vi "Keithley24XX_SR830_PPMS6000_4Probe_Resistance_Measurement - MasterSlave.vi"() -> ()   [LabVIEW 2019]
uses:
  <instrlib>/Stanford Research 830/Public/Data/Read (All Parameters).vi
  <instrlib>/Keithley 24XX/Public/Data/Read (Single Point).vi
  <instrlib>/Keithley 24XX/Keithley 24XX.lvlib
  <instrlib>/Stanford Research 830/Stanford Research 830.lvlib
panel:
  in  "Temperature Control":enum32{"XY Graph", "Waveform (Time)"}(tab)
  out "Temp vs Time : XYGraph 3":cluster{"Y":dbl[], "Y":dbl[]}[](graph)
  out "Temp vs Time: TimeGraph 3":cluster{dbl, "Theta-Value":dbl}[](graph)
  in  "PPMS Temp GPIB address":string="15"
  in  "Daugher Theta vs Vg":enum32{"XY Graph", "Waveform (Time)"}(tab)
  out "Parent Theta vs Vg : XYGraph 2":cluster{"Y":dbl[], "Y":dbl[]}[](graph)
  out "Parent: Theta vs Vg : TimeGraph 2":cluster{dbl, "Theta-Value":dbl}[](graph)
  in  "Daughter R vs Vg 2":enum32{"XY Graph", "Waveform (Time)"}(tab)
  out "Daughter Resistance vs Vg : XYGraph 2":cluster{"Y":dbl[], "Y":dbl[]}[](graph)
  out "Daughter: R vs Vg : TimeGraph 2":cluster{dbl, dbl}[](graph)
  out "dup path 2":path
  in  "<File Name>.txt (Don't add extension) 2":string
  in  "Data Save Path: Daughter":path=path "C:/Users/labpc/Documents/ProbeStation Users Data"
  in  "Sensitivity (Initial Value) 2":i16(ring)=17 items=["Auto Gain"=-1, "2 nV/fA"=0, "5 nV/fA"=1, "10 nV/fA"=2, "20 nV/fA"=3, "50 nV/fA"=4, "100 nV/fA"=5, "200 nV/fA"=6, "500 nV/fA"=7, "1 uV/pA"=8, "2 uV/pA"=9, "5 uV/pA"=10, "10 uV/pA"=11, "20 uV/pA"=12, "50 uV/pA"=13, "100 uV/pA"=14, "200 uV/pA"=15, "500 uV/pA"=16, "1 mV/nA"=17, "2 mV/nA"=18, "5 mV/nA"=19, "10 mV/nA"=20, "20 mV/nA"=21, "50 mV/nA"=22, "100 mV/nA"=23, "200 mV/nA"=24, "500 mV/mA"=25, "1 V/uA"=26]
  in  "Dynamic Reserve (-1 = Auto) 2":i16(ring)=1 items=["Auto Reserve"=-1, "High Reserve"=0, "Normal"=1, "Low Noise"=2]
  in  "Input Connection (0: Single-Ended Voltage)  2":u16(ring)=1 items=["Single-Ended Voltage", "Differential Voltage", "1 MOhm Current Gain", "100 MOhm Current Gain"]
  out "Input Coupling (0: AC) 2":u16(ring) items=["AC", "DC"]
  in  "Time Constant (8: 100ms) 2":u16(ring)=11 items=["10 us", "30 us", "100 us", "300 us", "1 ms", "3 ms", "10 ms", "30 ms", "100 ms", "300 ms", "1 s", "3 s", "10 s", "30 s", "100 s", "300 s", "1 ks", "3 ks", "10 ks", "30 ks"]
  in  "SR830 VISA resource name 2":refnum<visa-resource-name>="GPIB0::8::INSTR"
  in  "Trigger Source (0: Start Feature Off, 1: On)  - Data":u16(ring)=1 items=["Internal", "External"]
  out "Manual Phase (0 Degree) 2":dbl
  out "Detection Harmonic Number 2":dbl=1.0
  out "External Reference Trigger (0: Sine Zero Crossing)  2":u16(ring) items=["Sine Zero Crossing", "TTL Rising Edge", "TTL Falling Edge"]
  in  "Internal Reference Frequency (1000 Hz) 2":dbl=17.0
  in  "Reference Source (1: Internal) 2":u16(ring) items=["External", "Internal"]
  in  "Sine Output Amplitude (V) 2":dbl=1.0
  out "Gate\nVoltage":sgl
  out "Status":sgl
  out "Leakage \nCurrent":sgl
  out "dup path":path
  in  "<File Name>.txt (Don't add extension)":string
  in  "Data Save Path: Source":path=path "C:/Users/labpc/Documents/ProbeStation Users Data"
  in  "I_leak vs Vg":enum32{"XY Graph", "Waveform (Time)"}(tab)
  out "I_leak vs Vg : XYGraph":cluster{"Y":dbl[], "Y":dbl[]}[](graph)
  out "I_leak vs Vg : TimeGraph":cluster{dbl, "Current":sgl}[](graph)
  in  "Gate Voltage\nInitial (V)":dbl
  out "Gate Voltage\nTraversal Direction":enum16{"Upward", "Downward"}(ring)
  in  "Series Resistance \n(Apparatus Constant)":dbl=10000000.0
  in  "stop":bool
  out "Max/Min(-) \nGate Voltage (V)":dbl=80.0
  in  "Gate Voltage \nStep Size (V)":dbl=0.1
  in  "High Gate \nVoltage (V)":dbl
  in  "Low Gate \nVoltage (V)":dbl
  out "Compliance\n Level (A)":dbl=0.1
  in  "Parent Theta vs Vg":enum32{"XY Graph", "Waveform (Time)"}(tab)
  out "Parent Theta vs Vg : XYGraph":cluster{"Y":dbl[], "Y":dbl[]}[](graph)
  out "Parent: Theta vs Vg : TimeGraph":cluster{dbl, "Theta-Value":dbl}[](graph)
  in  "Parent R vs Vg":enum32{"XY Graph", "Waveform (Time)"}(tab)
  out "Parent Resistance vs Vg : XYGraph":cluster{"Y":dbl[], "Y":dbl[]}[](graph)
  out "Parent: R vs Vg : TimeGraph":cluster{dbl, dbl}[](graph)
  in  "Sensitivity (Initial Value)":i16(ring)=17 items=["Auto Gain"=-1, "2 nV/fA"=0, "5 nV/fA"=1, "10 nV/fA"=2, "20 nV/fA"=3, "50 nV/fA"=4, "100 nV/fA"=5, "200 nV/fA"=6, "500 nV/fA"=7, "1 uV/pA"=8, "2 uV/pA"=9, "5 uV/pA"=10, "10 uV/pA"=11, "20 uV/pA"=12, "50 uV/pA"=13, "100 uV/pA"=14, "200 uV/pA"=15, "500 uV/pA"=16, "1 mV/nA"=17, "2 mV/nA"=18, "5 mV/nA"=19, "10 mV/nA"=20, "20 mV/nA"=21, "50 mV/nA"=22, "100 mV/nA"=23, "200 mV/nA"=24, "500 mV/mA"=25, "1 V/uA"=26]
  in  "Dynamic Reserve (-1 = Auto)":i16(ring)=1 items=["Auto Reserve"=-1, "High Reserve"=0, "Normal"=1, "Low Noise"=2]
  in  "Input Connection (0: Single-Ended Voltage)":u16(ring)=1 items=["Single-Ended Voltage", "Differential Voltage", "1 MOhm Current Gain", "100 MOhm Current Gain"]
  out "Input Coupling (0: AC)":u16(ring) items=["AC", "DC"]
  in  "Time Constant (8: 100ms)":u16(ring)=11 items=["10 us", "30 us", "100 us", "300 us", "1 ms", "3 ms", "10 ms", "30 ms", "100 ms", "300 ms", "1 s", "3 s", "10 s", "30 s", "100 s", "300 s", "1 ks", "3 ks", "10 ks", "30 ks"]
  in  "SR830 VISA resource name":refnum<visa-resource-name>="GPIB0::10::INSTR"
  in  "Trigger Source (0: Internal)":u16(ring) items=["Internal", "External"]
  out "Manual Phase (0 Degree)":dbl
  out "Detection Harmonic Number":dbl=1.0
  out "External Reference Trigger (0: Sine Zero Crossing)":u16(ring) items=["Sine Zero Crossing", "TTL Rising Edge", "TTL Falling Edge"]
  in  "Internal Reference Frequency (1000 Hz)":dbl=17.0
  in  "Reference Source (1: Internal)":u16(ring)=1 items=["External", "Internal"]
  in  "Sine Output Amplitude (V)":dbl=1.0
  in  "Keithley24XX VISA resource name":refnum<visa-resource-name>="GPIB0::23::INSTR" caption="Keithley 24XX VISA resource name"
  out "Internal \nMeasurement\nTime":u32
  # "PPMS (QD_6000)"
  # "MAKE SURE THE SOURCE METER IS ON TO ENSURE NO UNINTENDED JUMPS. PROGRAM WILL KEEP SOURCE METER ON ONCE RUN."
  # "SR830 Lock In Amplifier  2 - Daughter"
  # "SR830 Lock In Amplifier  1 - Sourcing"
  # "Keithley 2400 SourceMeter"
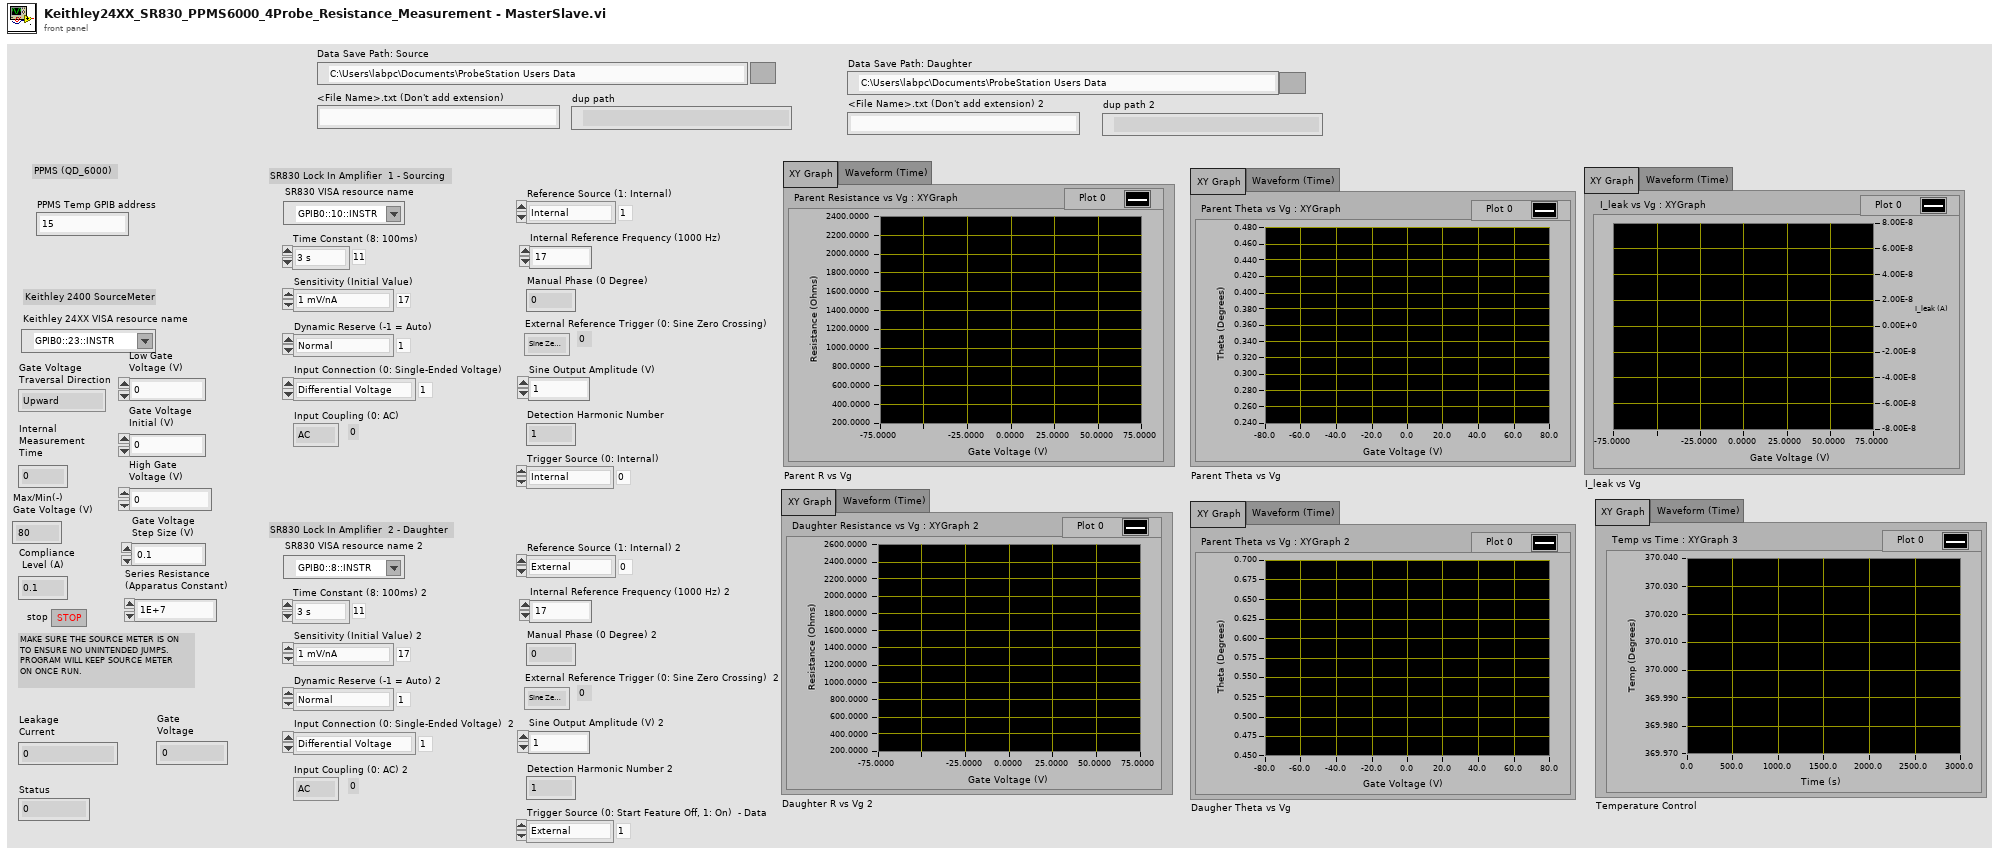
[diagram p1: front panel]
types:
  T1 = enum16{"open", "replace", "create", "open or create", "replace or create", "replace or create with confirmation"}
  T2 = cluster{"Baud Rate":u32, "Parity":u16, "Data Bits":u16, "Stop Bits":u16, "Flow Control":u16}
  T3 = cluster{"X-Value":dbl, "Y-Value":dbl, "R-Value":dbl, "Theta-Value":dbl, "Aux In 1 Value":dbl, "Aux In 2 Value":dbl, "Aux In 3 Value":dbl, "Aux In 4 Value":dbl, "Reference Frequency":dbl, "Channel 1 Display":dbl, "Channel 2 Display":dbl}
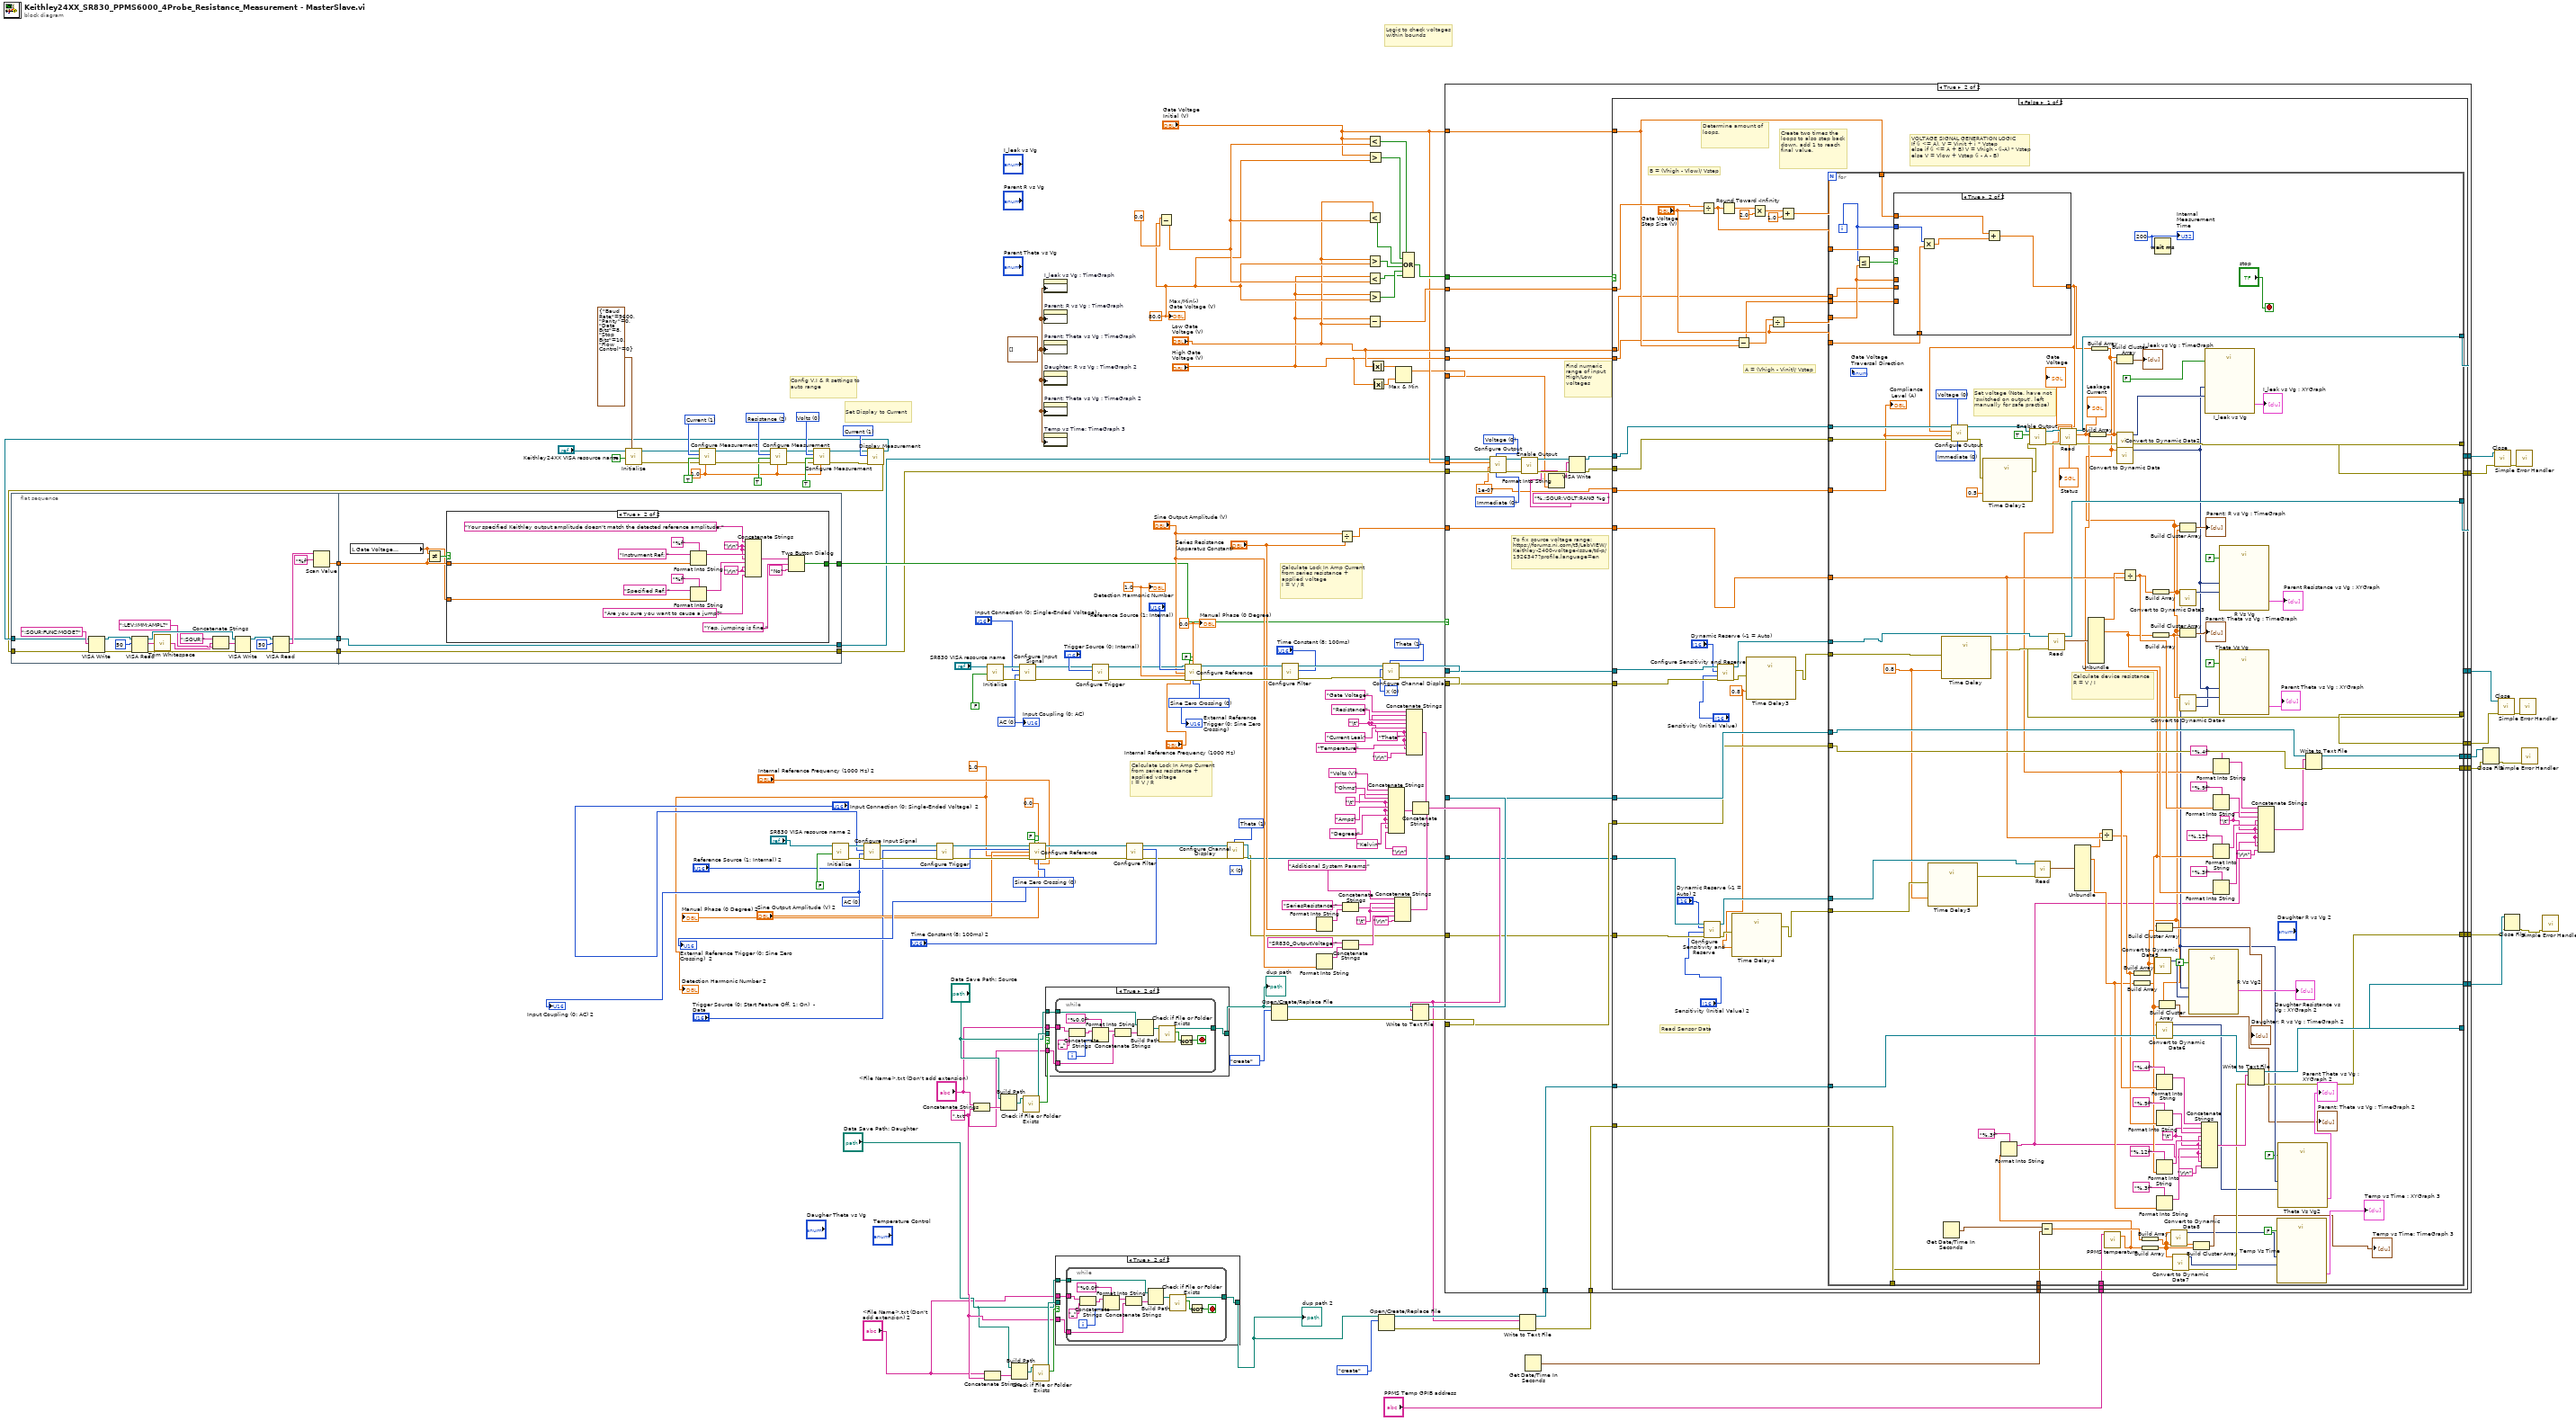
[diagram p0: block diagram]
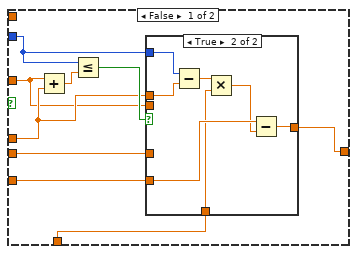
[diagram p4: hidden frame]
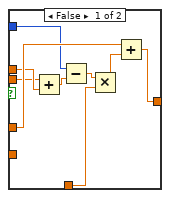
[diagram p5: hidden frame]
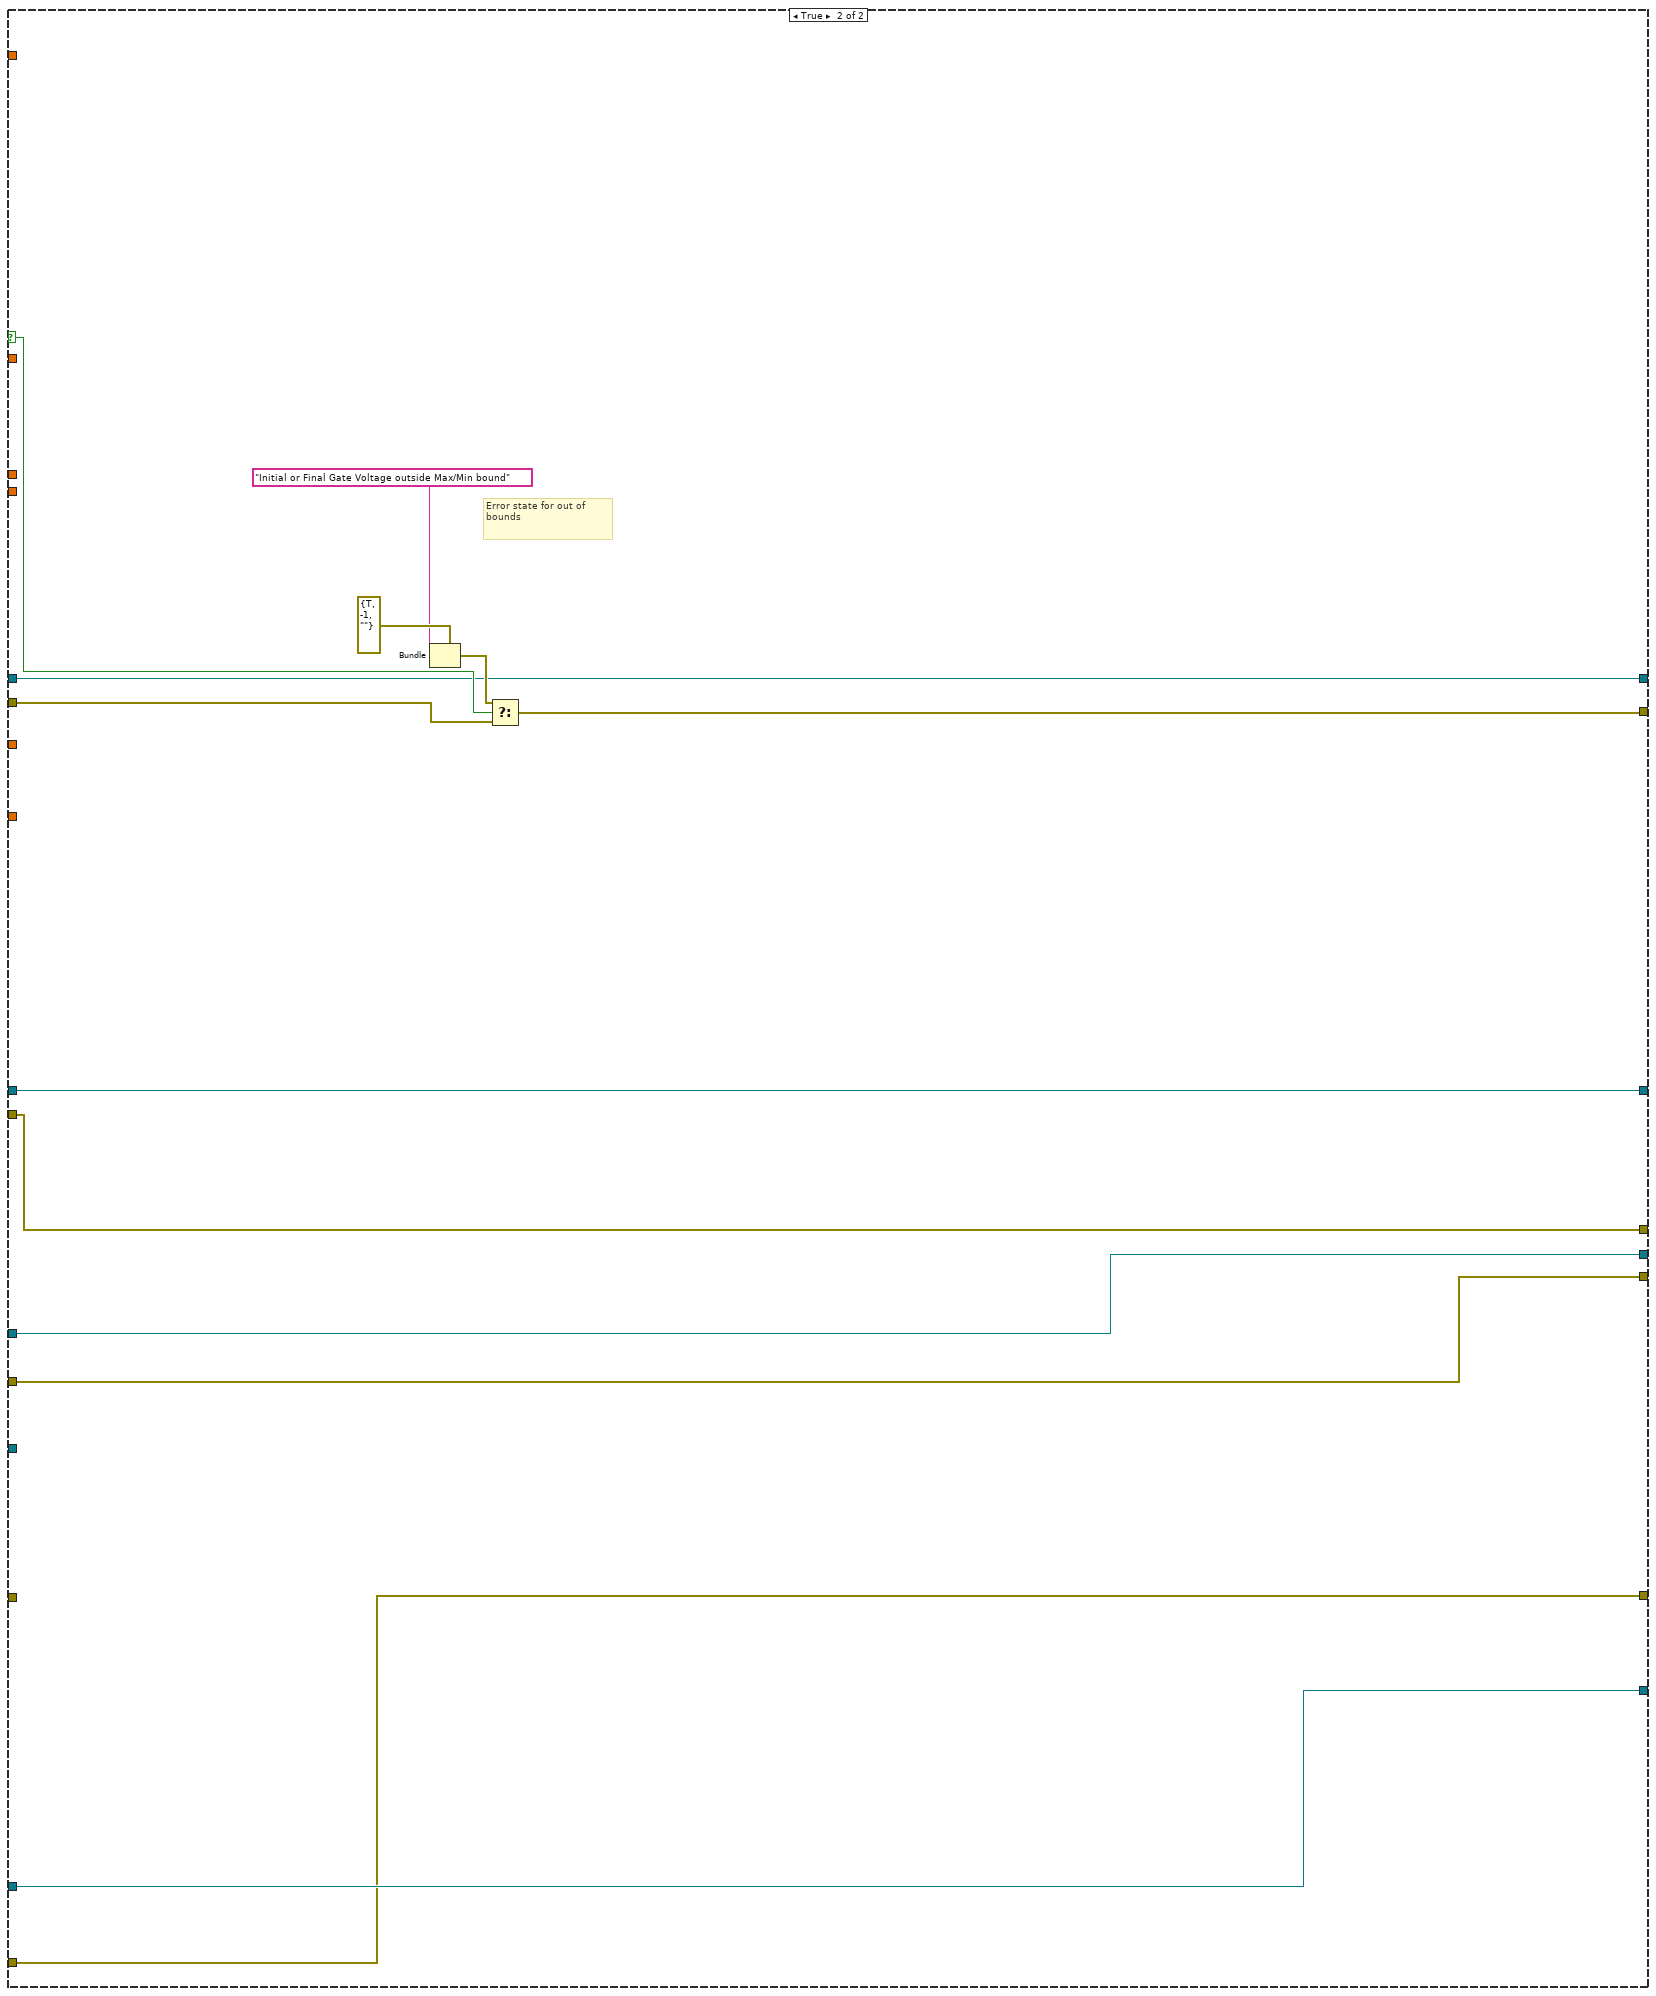
[diagram p6: hidden frame]
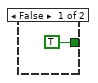
[diagram p7: hidden frame]
diagram:
  w7 = cluster{dbl, "Theta-Value":dbl}[] [] ("History Data")
  w12 = 0.0 ("Manual Phase (0 Degree)")
  w10 = 1.0 ("Detection Harmonic Number (1)")
  w26 = u16 0 items=["Sine Zero Crossing", "TTL Rising Edge", "TTL Falling Edge"] ("External Reference Trigger (0: Sine Zero Crossing)")
  w11 = u16 0 items=["AC", "DC"] ("Input Coupling (0: AC)")
  (unwired) u16 0 items=["X", "R", "X Noise", "Aux In 1", "Aux In 2"] ("Channel 1 Display (0: X)")
  w39 = u16 1 items=["Y", "Theta", "Y Noise", "Aux In 3", "Aux In 4"] ("Channel 2 Display  (0: Y)")
  w70 = "\t"
  w1 = "\t"
  w5 = "\t"
  w48 = ".txt"
  w104 = 1.0 ("Manual Range (1.0)")
  w125 = 0.0 ("Manual Phase (0 Degree)")
  w126 = 1.0 ("Detection Harmonic Number (1)")
  w127 = u16 0 items=["Sine Zero Crossing", "TTL Rising Edge", "TTL Falling Edge"] ("External Reference Trigger (0: Sine Zero Crossing)")
  w131 = u16 0 items=["AC", "DC"] ("Input Coupling (0: AC)")
  w116 = u16 0 items=["X", "R", "X Noise", "Aux In 1", "Aux In 2"] ("Channel 1 Display (0: X)")
  w141 = u16 1 items=["Y", "Theta", "Y Noise", "Aux In 3", "Aux In 4"] ("Channel 2 Display  (0: Y)")
  w146 = u16 1 items=["Voltage", "Current", "Resistance"] ("Displayed Measurement (0: Voltage)")
  w155 = u16 2 items=["Volts", "Current", "Resistance"] ("Function (0: Volts)")
  w159 = u16 1 items=["Volts", "Current", "Resistance"] ("Function (0: Volts)")
  w105 = 80.0
  w165 = u16 0 items=["Volts", "Current", "Resistance"] ("Function (0: Volts)")
  # "Calculate Lock In Amp Current from series resistance + applied voltage\nI = V / R"
  # "Logic to check voltages within bounds"
  # "Calculate Lock In Amp Current from series resistance + applied voltage\nI = V / R"
  # "Set Display to Current"
  # "Config V,I & R settings to auto range"
  n1 = flat-sequence {
    tunnel: [w169] -> w62
    tunnel: [w170] -> w61
    tunnel: [w171] -> w60
    tunnel: w59 -> [w168]
    tunnel: w58 -> [w167]
    tunnel: w62 -> [w190]
    tunnel: w61 -> [w189]
    tunnel: w60 -> [w193]
    tunnel: [w190] -> w54
    tunnel: [w189] -> w56
    tunnel: [w188] -> w57
    frame #0 {
      n2 = VISA Write(VISA resource name=w168, write buffer=":SOUR:FUNC:MODE?", error in (no error)=w167) -> (VISA resource name out=w184:refnum<visa-resource-name>, error out=w187:errorcluster)  [unwired: 1 out]
      n3 = VISA Read(VISA resource name=w184, byte count=u32 50, error in (no error)=w187) -> (VISA resource name out=w179:refnum<visa-resource-name>, read buffer=w173:string, error out=w180:errorcluster)  [unwired: 1 out]
      n4 = call <vilib>:"Trim Whitespace.vi"("string"=w173) -> ("trimmed string"=w172:string)  [unwired: 1 in]
      n5 = Concatenate Strings(":SOUR:" ("string"), w172, ":LEV:IMM:AMPL?" ("string")) -> (w176:string)
      n6 = VISA Write(VISA resource name=w179, write buffer=w176, error in (no error)=w180) -> (VISA resource name out=w181:refnum<visa-resource-name>, error out=w183:errorcluster)  [unwired: 1 out]
      n7 = VISA Read(VISA resource name=w181, byte count=u32 50, error in (no error)=w183) -> (VISA resource name out=w169:refnum<visa-resource-name>, read buffer=w174:string, error out=w170:errorcluster)  [unwired: 1 out]
      n8 = Scan Value(string=w174, format string="%f") -> (value=w171:dbl)  [unwired: 1 in, 1 out]
    }
    frame #1 {
      n9 = local read "Gate Voltage\nInitial (V)"() -> (w191:dbl)
      n10 = Not Equal?(x=w191, y=w193) -> (x != y?=w192:bool)
      n11 = case shown="True" w192 {
        tunnel: [TRUE ("T button?") w201] -> w188
        tunnel: w193 -> [_ w196]
        tunnel: w191 -> [_ w195]
        frame False {
        }
        frame True {
          w199 = "\r\n"
          w197 = "\r\n"
          n12 = Format Into String(format string="%f", initial string="Instrument Ref: ", w196) -> (resulting string=w203:string)  [unwired: 1 in, 1 out]
          n13 = Format Into String(format string="%f", initial string="Specified Ref: ", w195) -> (resulting string=w202:string)  [unwired: 1 in, 1 out]
          n14 = Concatenate Strings("Your specified Keithley output amplitude doesn't match the detected reference amplitude." ("message"), w197, w197, w203, w197, w202, w199, w199, "Are you sure you want to cause a jump?" ("string")) -> (w208:string)
          n15 = Two Button Dialog(message=w208, 1:"No" ("F button name (\"Cancel\")"), 2:"Yep, jumping is fine." ("T button name (\"OK\")")) -> (T button?=w201:bool)
        }
      }
    }
  }
  n16 = call <instrlib>:"Initialize.vi"("Serial Configuration"=T2 {"Baud Rate"=9600, "Parity"=0, "Data Bits"=8, "Stop Bits"=10, "Flow Control"=0}, "Reset (True)"=FALSE, "VISA resource name"="Keithley24XX VISA resource name") -> ("error out"=w150:errorcluster, "VISA resource name out"=w151:refnum<visa-resource-name>)  [unwired: 7 in]
  n17 = call <instrlib>:"Configure Measurement.vi"("Manual Range (1.0)"=w104, "error in (no error)"=w150, "Enable Auto Range (T:Enable)"=TRUE, "Function (0: Volts)"=w159, "VISA resource name"=w151) -> ("error out"=w157:errorcluster, "VISA resource name out"=w152:refnum<visa-resource-name>)  [unwired: 5 in]
  n18 = call <instrlib>:"Configure Measurement.vi"("Manual Range (1.0)"=w104, "error in (no error)"=w157, "Enable Auto Range (T:Enable)"=TRUE, "Function (0: Volts)"=w155, "VISA resource name"=w152) -> ("error out"=w154:errorcluster, "VISA resource name out"=w153:refnum<visa-resource-name>)  [unwired: 5 in]
  n19 = call <instrlib>:"Configure Measurement.vi"("Manual Range (1.0)"=w104, "error in (no error)"=w154, "Enable Auto Range (T:Enable)"=TRUE, "Function (0: Volts)"=w165, "VISA resource name"=w153) -> ("error out"=w144:errorcluster, "VISA resource name out"=w145:refnum<visa-resource-name>)  [unwired: 5 in]
  n20 = call <instrlib>:"Initialize.vi"("Reset (True)"=FALSE, "VISA resource name"="SR830 VISA resource name 2") -> ("error out"=w37:errorcluster, "VISA resource name out"=w38:refnum<visa-resource-name>)  [unwired: 8 in]
  n21 = call <instrlib>:"Configure Input Signal.vi"("error in (no error)"=w37, "Input Coupling (0: AC)"=w11, "Input Connection (0: Single-Ended Voltage)"="Input Connection (0: Single-Ended Voltage)  2", "VISA resource name"=w38) -> ("error out"=w33:errorcluster, "VISA resource name out"=w34:refnum<visa-resource-name>)  [unwired: 6 in]
  n22 = call <instrlib>:"Display Measurement.vi"("error in (no error)"=w144, "Displayed Measurement (0: Voltage)"=w146, "VISA resource name"=w145) -> ("error out"=w58:errorcluster, "VISA resource name out"=w59:refnum<visa-resource-name>)  [unwired: 7 in]
  n23 = call <instrlib>:"Configure Trigger.vi"("error in (no error)"=w33, "Trigger Source (0: Internal)"="Trigger Source (0: Start Feature Off, 1: On)  - Data", "VISA resource name"=w34) -> ("error out"=w31:errorcluster, "VISA resource name out"=w32:refnum<visa-resource-name>)  [unwired: 7 in]
  n24 = Concatenate Strings("<File Name>.txt (Don't add extension)", w48) -> (w103:string)
  n25 = Concatenate Strings("<File Name>.txt (Don't add extension) 2", w48) -> (w52:string)
  n26 = call <instrlib>:"Initialize.vi"("Reset (True)"=FALSE, "VISA resource name"="SR830 VISA resource name") -> ("error out"=w138:errorcluster, "VISA resource name out"=w139:refnum<visa-resource-name>)  [unwired: 8 in]
  n27 = Build Path(base path="Data Save Path: Source", name or relative path=w103) -> (appended path=w102:path)
  n28 = Build Path(base path="Data Save Path: Daughter", name or relative path=w52) -> (appended path=w51:path)
  n29 = call <instrlib>:"Configure Input Signal.vi"("error in (no error)"=w138, "Input Coupling (0: AC)"=w131, "Input Connection (0: Single-Ended Voltage)"="Input Connection (0: Single-Ended Voltage)", "VISA resource name"=w139) -> ("error out"=w122:errorcluster, "VISA resource name out"=w123:refnum<visa-resource-name>)  [unwired: 6 in]
  n30 = call <vilib>:"Check if File or Folder Exists.vi"("path"=w102) -> ("file or folder exists?"=w101:bool, "dup path"=w100:path)  [unwired: 8 in, 1 out]
  n31 = call <instrlib>:"Configure Reference.vi"("VISA resource name"=w32, "Auto Phase (T: Enabled)"=FALSE, "Manual Phase (0 Degree)"=w12, "Reference Source (1: Internal)"="Reference Source (1: Internal) 2", "Sine Output Amplitude (1 V)"="Sine Output Amplitude (V) 2", "Detection Harmonic Number (1)"=w10, "error in (no error)"=w31, "Internal Reference Frequency (1000 Hz)"="Internal Reference Frequency (1000 Hz) 2", "External Reference Trigger (0: Sine Zero Crossing)"=w26) -> ("VISA resource name out"=w35:refnum<visa-resource-name>, "error out"=w36:errorcluster)  [unwired: 5 in]
  n32 = call <vilib>:"Check if File or Folder Exists.vi"("path"=w51) -> ("file or folder exists?"=w50:bool, "dup path"=w49:path)  [unwired: 8 in, 1 out]
  n33 = property on="I_leak vs Vg : TimeGraph" class="WFChart (strict)"("History Data"=w7) -> ()  [unwired: 2 in, 2 out]
  n34 = property on="Parent: R vs Vg : TimeGraph" class="WFChart (strict)"("History Data"=w7) -> ()  [unwired: 2 in, 2 out]
  n35 = property on="Parent: Theta vs Vg : TimeGraph" class="WFChart (strict)"("History Data"=w7) -> ()  [unwired: 2 in, 2 out]
  n36 = property on="Daughter: R vs Vg : TimeGraph 2" class="WFChart (strict)"("History Data"=w7) -> ()  [unwired: 2 in, 2 out]
  n37 = property on="Parent: Theta vs Vg : TimeGraph 2" class="WFChart (strict)"("History Data"=w7) -> ()  [unwired: 2 in, 2 out]
  n38 = property on="Temp vs Time: TimeGraph 3" class="WFChart (strict)"("History Data"=w7) -> ()  [unwired: 2 in, 2 out]
  n39 = case shown="True" w101 {
    tunnel: [w211 w212] -> w95
    tunnel: w100 -> [w211 _]
    tunnel: "Data Save Path: Source" -> [_ w213]
    tunnel: "<File Name>.txt (Don't add extension)" -> [_ w215]
    tunnel: w48 -> [_ w214]
    frame False {
    }
    frame True {
      n40 = while {
        tunnel: w215 -> [w218]
        tunnel: w214 -> [w223]
        tunnel: w213 -> [w221]
        tunnel: [w219] -> w212
        i -> [w225]
        stop <- w227 stop-if-true
        n41 = Concatenate Strings(w218, "_" ("string")) -> (w217:string)
        n42 = Format Into String(format string="%0.0f", initial string=w217, w225) -> (resulting string=w224:string)  [unwired: 1 in, 1 out]
        n43 = Concatenate Strings(w224, w223) -> (w222:string)
        n44 = Build Path(base path=w221, name or relative path=w222) -> (appended path=w220:path)
        n45 = call <vilib>:"Check if File or Folder Exists.vi"("path"=w220) -> ("file or folder exists?"=w228:bool, "dup path"=w219:path)  [unwired: 8 in, 1 out]
        n46 = Not(x=w228) -> (.not. x?=w227:bool)
      }
    }
  }
  "dup path" <- w95
  n47 = case shown="True" w50 {
    tunnel: [w229 w230] -> w42
    tunnel: w49 -> [w229 _]
    tunnel: "Data Save Path: Daughter" -> [_ w231]
    tunnel: "<File Name>.txt (Don't add extension) 2" -> [_ w233]
    tunnel: w48 -> [_ w232]
    frame False {
    }
    frame True {
      n48 = while {
        tunnel: w233 -> [w236]
        tunnel: w232 -> [w241]
        tunnel: w231 -> [w239]
        tunnel: [w237] -> w230
        i -> [w243]
        stop <- w245 stop-if-true
        n49 = Concatenate Strings(w236, "_" ("string")) -> (w235:string)
        n50 = Format Into String(format string="%0.0f", initial string=w235, w243) -> (resulting string=w242:string)  [unwired: 1 in, 1 out]
        n51 = Concatenate Strings(w242, w241) -> (w240:string)
        n52 = Build Path(base path=w239, name or relative path=w240) -> (appended path=w238:path)
        n53 = call <vilib>:"Check if File or Folder Exists.vi"("path"=w238) -> ("file or folder exists?"=w246:bool, "dup path"=w237:path)  [unwired: 8 in, 1 out]
        n54 = Not(x=w246) -> (.not. x?=w245:bool)
      }
    }
  }
  "dup path 2" <- w42
  n55 = call <instrlib>:"Configure Trigger.vi"("error in (no error)"=w122, "Trigger Source (0: Internal)"="Trigger Source (0: Internal)", "VISA resource name"=w123) -> ("error out"=w120:errorcluster, "VISA resource name out"=w121:refnum<visa-resource-name>)  [unwired: 7 in]
  n56 = call <instrlib>:"Configure Filter.vi"("error in (no error)"=w36, "Time Constant (8: 100ms)"="Time Constant (8: 100ms) 2", "VISA resource name"=w35) -> ("error out"=w19:errorcluster, "VISA resource name out"=w20:refnum<visa-resource-name>)  [unwired: 7 in]
  n57 = Subtract(x=0.0, y=w105) -> (x-y=w110:dbl)
  n58 = call <instrlib>:"Configure Reference.vi"("VISA resource name"=w121, "Auto Phase (T: Enabled)"=FALSE, "Manual Phase (0 Degree)"=w125, "Reference Source (1: Internal)"="Reference Source (1: Internal)", "Sine Output Amplitude (1 V)"="Sine Output Amplitude (V)", "Detection Harmonic Number (1)"=w126, "error in (no error)"=w120, "Internal Reference Frequency (1000 Hz)"="Internal Reference Frequency (1000 Hz)", "External Reference Trigger (0: Sine Zero Crossing)"=w127) -> ("VISA resource name out"=w128:refnum<visa-resource-name>, "error out"=w129:errorcluster)  [unwired: 5 in]
  n59 = call <instrlib>:"Configure Channel Display.vi"("Channel 2 Display  (0: Y)"=w39, "error in (no error)"=w19, "VISA resource name"=w20) -> ("error out"=w17:errorcluster, "VISA resource name out"=w18:refnum<visa-resource-name>)  [unwired: 7 in]
  n60 = Open/Create/Replace File(file path (use dialog)=w95, operation (0:open)=T1."create") -> (refnum out=w96:refnum<file>, error out=w94:errorcluster)  [unwired: 4 in, 1 out]
  n61 = call <instrlib>:"Configure Filter.vi"("error in (no error)"=w129, "Time Constant (8: 100ms)"="Time Constant (8: 100ms)", "VISA resource name"=w128) -> ("error out"=w148:errorcluster, "VISA resource name out"=w147:refnum<visa-resource-name>)  [unwired: 7 in]
  n62 = Format Into String("Series Resistance \n(Apparatus Constant)") -> (resulting string=w88:string)  [unwired: 3 in, 1 out]
  n63 = Format Into String("Sine Output Amplitude (V)") -> (resulting string=w87:string)  [unwired: 3 in, 1 out]
  n64 = Divide(x="Sine Output Amplitude (V)", y="Series Resistance \n(Apparatus Constant)") -> (x/y=w119:dbl)
  n65 = Concatenate Strings("SeriesResistance:" ("string"), w88) -> (w69:string)
  n66 = Concatenate Strings("SR830_OutputVoltage:" ("string"), w87) -> (w68:string)
  n67 = Less?(x="Gate Voltage\nInitial (V)", y=w110) -> (x < y?=w108:bool)
  n68 = Less?(x="Low Gate \nVoltage (V)", y=w110) -> (x < y?=w114:bool)
  n69 = Greater?(x="Low Gate \nVoltage (V)", y=w105) -> (0:w113:bool)
  n70 = Less?(x="High Gate \nVoltage (V)", y=w110) -> (x < y?=w111:bool)
  n71 = Greater?(x="High Gate \nVoltage (V)", y=w105) -> (0:w112:bool)
  n72 = Subtract(x="High Gate \nVoltage (V)", y="Low Gate \nVoltage (V)") -> (x-y=w106:dbl)
  n73 = Greater?(x="Gate Voltage\nInitial (V)", y=w105) -> (0:w109:bool)
  n74 = Absolute Value(x="Low Gate \nVoltage (V)") -> (abs(x)=w66:dbl)
  n75 = Absolute Value(x="High Gate \nVoltage (V)") -> (abs(x)=w65:dbl)
  n76 = Open/Create/Replace File(file path (use dialog)=w42, operation (0:open)=T1."create") -> (refnum out=w44:refnum<file>, error out=w43:errorcluster)  [unwired: 4 in, 1 out]
  n77 = call <instrlib>:"Configure Channel Display.vi"("Channel 2 Display  (0: Y)"=w141, "error in (no error)"=w148, "Channel 1 Display (0: X)"=w116, "VISA resource name"=w147) -> ("error out"=w136:errorcluster, "VISA resource name out"=w137:refnum<visa-resource-name>)  [unwired: 6 in]
  n78 = Concatenate Strings("Volts (V)" ("string"), w1, "Ohms" ("string"), w1, "Amps" ("string"), w1, "Degrees" ("string"), w1, "Kelvin" ("string"), w1, "\r\n") -> (w81:string)
  n79 = Concatenate Strings("Additional System Params:" ("string"), w70, w69, w70, w68, "\r\n") -> (w71:string)
  n80 = Max & Min(x=w66, y=w65) -> (max(x,y)=w53:dbl)  [unwired: 1 out]
  n81 = Compound Arithmetic op=OR(w108, w109, w114, w113, w112, w111) -> (w107:bool)
  n82 = Concatenate Strings("Gate Voltage" ("string"), w5, "Resistance" ("string"), w5, "Current Leak" ("string"), w5, "Theta" ("string"), w5, "Temperature" ("string"), w5, "\r\n") -> (w82:string)
  n83 = Concatenate Strings(w82, w81, w71) -> (w41:string)
  n84 = Write to Text File(file (use dialog)=w96, text=w41, error in=w94) -> (refnum out=w92:refnum<file>, error out=w91:errorcluster)  [unwired: 1 in, 1 out]
  n85 = Write to Text File(file (use dialog)=w44, text=w41, error in=w43) -> (refnum out=w24:refnum<file>, error out=w22:errorcluster)  [unwired: 1 in, 1 out]
  n86 = Get Date/Time In Seconds() -> (seconds since 1Jan1904=w8:timestamp)
  n87 = case shown="True" w57 {
    tunnel: [w254 w293] -> w163
    tunnel: [w253 w292] -> w162
    tunnel: w137 -> [w252 w291]
    tunnel: w136 -> [w251 w290]
    tunnel: [w252 w289] -> w135
    tunnel: [w251 w288] -> w134
    tunnel: w119 -> [_ w287]
    tunnel: w107 -> [_ w286]
    tunnel: w106 -> [_ w285]
    tunnel: w92 -> [w250 w284]
    tunnel: w91 -> [w249 w283]
    tunnel: [w250 w282] -> w90
    tunnel: [w249 w281] -> w89
    tunnel: "Low Gate \nVoltage (V)" -> [_ w280]
    tunnel: "High Gate \nVoltage (V)" -> [_ w279]
    tunnel: "Gate Voltage\nInitial (V)" -> [_ w278]
    tunnel: w56 -> [w253 w270]
    tunnel: "Gate Voltage\nInitial (V)" -> [_ w269]
    tunnel: w54 -> [w254 w268]
    tunnel: w53 -> [_ w266]
    tunnel: [w248 w262] -> w25
    tunnel: w24 -> [w248 w261]
    tunnel: [w247 w260] -> w23
    tunnel: w22 -> [w247 w259]
    tunnel: w18 -> [_ w258]
    tunnel: w17 -> [_ w257]
    tunnel: "PPMS Temp GPIB address" -> [_ w256]
    tunnel: w8 -> [_ w255]
    frame False {
    }
    frame True {
      w272 = u16 0 items=["Immediate", "Triggered"] ("Output Type  (0: Immediate)")
      w265 = 1e-07 ("Compliance  Level (0.1)")
      w271 = u16 0 items=["Voltage", "Current"] ("Source Mode  (0: Voltage)")
      # "Find numeric range of input High/Low voltages"
      # "To fix source voltage range:\nhttps://forums.ni.com/t5/LabVIEW/Keithley-2400-voltage-Issue/td-p/1926347?profile.language=en"
      n88 = call <instrlib>:"Configure Output.vi"("Output Type  (0: Immediate)"=w272, "Source Mode  (0: Voltage)"=w271, "error in (no error)"=w270, "Compliance  Level (0.1)"=w265, "Output Level (0)"=w269, "VISA resource name"=w268) -> ("error out"=w277:errorcluster, "VISA resource name out"=w276:refnum<visa-resource-name>)  [unwired: 4 in]
      n89 = call <instrlib>:"Enable Output.vi"("error in (no error)"=w277, "VISA resource name"=w276) -> ("error out"=w275:errorcluster, "VISA resource name out"=w274:refnum<visa-resource-name>)  [unwired: 8 in]
      n90 = Format Into String(format string="%.;SOUR:VOLT:RANG %g ", w266) -> (resulting string=w273:string)  [unwired: 2 in, 1 out]
      n91 = VISA Write(VISA resource name=w274, write buffer=w273, error in (no error)=w275) -> (VISA resource name out=w263:refnum<visa-resource-name>, error out=w264:errorcluster)  [unwired: 1 out]
      n92 = case shown="False" w286 {
        selector: w286 -> [_ w499]
        tunnel: w264 -> [w339 w498]
        tunnel: w263 -> [w309 w493]
        tunnel: [w338 w493] -> w293
        tunnel: [w337 w494] -> w292
        tunnel: w291 -> [w332 w492]
        tunnel: w290 -> [w333 w491]
        tunnel: [w335 w492] -> w289
        tunnel: [w334 w491] -> w288
        tunnel: w287 -> [w329 _]
        tunnel: w285 -> [w324 _]
        tunnel: w280 -> [w317 _]
        tunnel: w279 -> [w318 _]
        tunnel: w278 -> [w320 _]
        tunnel: w284 -> [w314 w490]
        tunnel: w283 -> [w313 w489]
        tunnel: [w312 w490] -> w282
        tunnel: [w311 w489] -> w281
        tunnel: w265 -> [w308 _]
        tunnel: [w307 w488] -> w262
        tunnel: w261 -> [w306 w488]
        tunnel: [w305 w487] -> w260
        tunnel: w259 -> [w304 w487]
        tunnel: w258 -> [w302 _]
        tunnel: w257 -> [w301 _]
        tunnel: w256 -> [w296 _]
        tunnel: w255 -> [w295 _]
        frame False {
          w297 = 0.8 ("Delay Time (s)")
          # "Read Sensor Data"
          # "VOLTAGE SIGNAL GENERATION LOGIC\nIf (i <= A), V = Vinit + i * Vstep\nelse if (i <= A + B) V = Vhigh - (i-A) * Vstep\nelse V = Vlow + Vstep (i - A - B)"
          # "B = (Vhigh - Vlow)/ Vstep"
          # "A = (Vhigh - Vinit)/ Vstep"
          # "Create two times the loops to also step back down, add 1 to reach final value."
          # "Determine amount of loops,"
          n93 = Divide(x=w324, y="Gate Voltage \nStep Size (V)") -> (x/y=w319:dbl)
          n94 = call <instrlib>:"Configure Sensitivity and Reserve.vi"("error in (no error)"=w301, "Sensitivity (-1: Auto gain)"="Sensitivity (Initial Value) 2", "Dynamic Reserve (-1: Auto Reserve)"="Dynamic Reserve (-1 = Auto) 2", "VISA resource name"=w302) -> ("error out"=w303:errorcluster, "VISA resource name out"=w300:refnum<visa-resource-name>)  [unwired: 6 in]
          n95 = call <instrlib>:"Configure Sensitivity and Reserve.vi"("error in (no error)"=w333, "Sensitivity (-1: Auto gain)"="Sensitivity (Initial Value)", "Dynamic Reserve (-1: Auto Reserve)"="Dynamic Reserve (-1 = Auto)", "VISA resource name"=w332) -> ("error out"=w315:errorcluster, "VISA resource name out"=w331:refnum<visa-resource-name>)  [unwired: 6 in]
          n96 = Round Toward -Infinity(1:w319) -> (0:w327:dbl)
          n97 = call "Time Delay4"("error in (no error)"=w303, "Delay Time (s)"=w297) -> ("error out"=w299:errorcluster)  [unwired: 9 in]
          n98 = Subtract(x=w318, y=w320) -> (x-y=w323:dbl)
          n99 = call "Time Delay3"("error in (no error)"=w315, "Delay Time (s)"=w297) -> ("error out"=w316:errorcluster)  [unwired: 9 in]
          n100 = Multiply(x=w327, y=2.0) -> (x*y=w326:dbl)
          n101 = Divide(x=w323, y="Gate Voltage \nStep Size (V)") -> (x/y=w321:dbl)
          n102 = Add(x=w326, y=1.0) -> (x+y=w325:dbl)
          n103 = for {
            N: w325 -> [_]
            tunnel: w309 -> [w452]
            tunnel: w339 -> [w418]
            tunnel: [w456] -> w338
            tunnel: [w455] -> w337
            tunnel: [w445] -> w335
            tunnel: [w446] -> w334
            tunnel: w331 -> [w400]
            tunnel: w316 -> [w401]
            tunnel: w329 -> [w389]
            tunnel: "Gate Voltage \nStep Size (V)" -> [w424]
            tunnel: w321 -> [w422]
            tunnel: w320 -> [w425]
            tunnel: w319 -> [w423]
            tunnel: w318 -> [w421]
            tunnel: w317 -> [w420]
            tunnel: w314 -> [w415]
            tunnel: w313 -> [w414]
            tunnel: [w413] -> w312
            tunnel: [w412] -> w311
            tunnel: w308 -> [w395]
            tunnel: [w377] -> w307
            tunnel: w306 -> [w378]
            tunnel: [w375] -> w305
            tunnel: w304 -> [w376]
            tunnel: w300 -> [w392]
            tunnel: w299 -> [w391]
            tunnel: w296 -> [w357]
            tunnel: w295 -> [w353]
            i -> [w399]
            stop <- "stop" stop-if-true
            w346 = "\t"
            w342 = "\t"
            w419 = u16 0 items=["Immediate", "Triggered"] ("Output Type  (0: Immediate)")
            w390 = 0.8 ("Delay Time (s)")
            w453 = u32 200 ("milliseconds to wait")
            w448 = u16 0 items=["Voltage", "Current"] ("Source Mode  (0: Voltage)")
            # "Calculate device resistance\nR = V / I"
            # "Set voltage (Note, have not 'switched on output', left manually for safe practise)"
            n104 = Less Or Equal?(x=w399, y=w422) -> (x <= y?=w426:bool)
            n105 = case shown="True" w426 {
              tunnel: [w463 w482] -> w374
              tunnel: w425 -> [_ w485]
              tunnel: w399 -> [w460 w486]
              tunnel: w424 -> [w461 w483]
              tunnel: w423 -> [w457 _]
              tunnel: w422 -> [w459 _]
              tunnel: w421 -> [w462 _]
              tunnel: w420 -> [w458 _]
              frame False {
                n106 = Add(x=w457, y=w459) -> (x+y=w464:dbl)
                n107 = Less Or Equal?(x=w460, y=w464) -> (x <= y?=w465:bool)
                n108 = case shown="True" w465 {
                  tunnel: [w471 w480] -> w463
                  tunnel: w462 -> [_ w481]
                  tunnel: w461 -> [w473 w478]
                  tunnel: w460 -> [w468 w477]
                  tunnel: w459 -> [w467 w476]
                  tunnel: w458 -> [w474 _]
                  tunnel: w457 -> [w466 _]
                  frame False {
                    n109 = Add(x=w466, y=w467) -> (x+y=w469:dbl)
                    n110 = Subtract(x=w468, y=w469) -> (x-y=w470:dbl)
                    n111 = Multiply(x=w470, y=w473) -> (x*y=w472:dbl)
                    n112 = Add(x=w474, y=w472) -> (x+y=w471:dbl)
                  }
                  frame True {
                    n113 = Subtract(x=w477, y=w476) -> (x-y=w479:dbl)
                    n114 = Multiply(x=w479, y=w478) -> (x*y=w475:dbl)
                    n115 = Subtract(x=w481, y=w475) -> (x-y=w480:dbl)
                  }
                }
              }
              frame True {
                n116 = Multiply(x=w486, y=w483) -> (x*y=w484:dbl)
                n117 = Add(x=w485, y=w484) -> (x+y=w482:dbl)
              }
            }
            n118 = call "Time Delay5"("error in (no error)"=w391, "Delay Time (s)"=w390) -> ("error out"=w393:errorcluster)  [unwired: 9 in]
            n119 = call "Time Delay"("error in (no error)"=w401, "Delay Time (s)"=w390) -> ("error out"=w442:errorcluster)  [unwired: 9 in]
            n120 = Get Date/Time In Seconds() -> (seconds since 1Jan1904=w354:timestamp)
            n121 = call <instrlib>:"Configure Output.vi"("Output Type  (0: Immediate)"=w419, "Source Mode  (0: Voltage)"=w448, "error in (no error)"=w418, "Compliance  Level (0.1)"=w395, "Output Level (0)"=w374, "VISA resource name"=w452) -> ("error out"=w417:errorcluster, "VISA resource name out"=w451:refnum<visa-resource-name>)  [unwired: 4 in]
            n122 = call "Time Delay2"("error in (no error)"=w417, "Delay Time (s)"=0.5) -> ("error out"=w416:errorcluster)  [unwired: 9 in]
            n123 = call <instrlib>:"Enable Output.vi"("error in (no error)"=w416, "Enable Output (T: Enable)"=TRUE, "VISA resource name"=w451) -> ("error out"=w450:errorcluster, "VISA resource name out"=w449:refnum<visa-resource-name>)  [unwired: 7 in]
            n124 = call-poly <instrlib>:"Read.vi"("error in (no error)"=w393, "VISA resource name"=w392) -> ("Parameter Values"=w394:T3)  [unwired: 7 in, 2 out]
            n125 = Subtract(x=w354, y=w353) -> (x-y=w352:dbl)
            n126 = call-poly <instrlib>:"Read.vi"("error in (no error)"=w442, "VISA resource name"=w400) -> ("error out"=w446:errorcluster, "Parameter Values"=w444:T3, "VISA resource name out"=w445:refnum<visa-resource-name>)  [unwired: 7 in]
            n127 = call-poly <instrlib>:"Read.vi"("VISA resource name"=w449, "error in (no error)"=w450) -> ("Voltage"=→"Gate\nVoltage":sgl, "VISA resource name out"=w456:refnum<visa-resource-name>, "Current"=w371:sgl, "Status"=→"Status":sgl, "error out"=w455:errorcluster)  [unwired: 7 in, 2 out]
            "Leakage \nCurrent" <- w371
            n128 = Unbundle(w394) -> ("X-Value"=w388:dbl, "Theta-Value"=w372:dbl)  [unwired: 9 out]
            n129 = Unbundle(w444) -> ("X-Value"=w443:dbl, "Theta-Value"=w405:dbl)  [unwired: 9 out]
            n130 = Build Array(w371) -> (w439:sgl[])
            n131 = Build Array(w374) -> (w363:dbl[])
            n132 = Divide(x=w388, y=w389) -> (x/y=w373:dbl)
            n133 = call <instrlib>:"PPMS temperature.vi"("GPIB address"=w357) -> ("Temperature (K)"=w344:dbl)  [unwired: 2 in, 1 out]
            n134 = Format Into String(format string="%.3f", w344) -> (resulting string=w341:string)  [unwired: 2 in, 1 out]
            n135 = Build Cluster Array(w363, w439) -> (→"I_leak vs Vg : TimeGraph":cluster{dbl, "Current":sgl}[])
            n136 = call "Convert to Dynamic Data2"("Array"=w439) -> ("Dynamic Data Type"=w438:dynamicdata)  [unwired: 3 in]
            n137 = call "Convert to Dynamic Data"("Array"=w363) -> ("Dynamic Data Type"=w366:dynamicdata)  [unwired: 3 in]
            n138 = Divide(x=w443, y=w389) -> (x/y=w406:dbl)
            n139 = Build Array(w373) -> (w368:dbl[])
            n140 = Build Array(w372) -> (w362:dbl[])
            n141 = Build Array(w352) -> (w351:dbl[])
            n142 = Build Array(w344) -> (w350:dbl[])
            n143 = Build Array(w406) -> (w437:dbl[])
            n144 = Build Array(w405) -> (w435:dbl[])
            n145 = Wait (ms)(milliseconds to wait=w453) -> ()  [unwired: 1 out]
            n146 = call "Convert to Dynamic Data5"("Array"=w368) -> ("Dynamic Data Type"=w367:dynamicdata)  [unwired: 3 in]
            n147 = Format Into String(format string="%.4f", w374) -> (resulting string=w387:string)  [unwired: 2 in, 1 out]
            n148 = Format Into String(format string="%.9f", w373) -> (resulting string=w386:string)  [unwired: 2 in, 1 out]
            n149 = Format Into String(format string="%.12f", w371) -> (resulting string=w385:string)  [unwired: 2 in, 1 out]
            n150 = Format Into String(format string="%.3f", w372) -> (resulting string=w384:string)  [unwired: 2 in, 1 out]
            n151 = Build Cluster Array(w363, w368) -> (→"Daughter: R vs Vg : TimeGraph 2":cluster{dbl, dbl}[])
            n152 = call "Convert to Dynamic Data6"("Array"=w362) -> ("Dynamic Data Type"=w365:dynamicdata)  [unwired: 3 in]
            n153 = Build Cluster Array(w363, w362) -> (→"Parent: Theta vs Vg : TimeGraph 2":cluster{dbl, "Theta-Value":dbl}[])
            n154 = call "Convert to Dynamic Data8"("Array"=w351) -> ("Dynamic Data Type"=w349:dynamicdata)  [unwired: 3 in]
            n155 = call "Convert to Dynamic Data7"("Array"=w350) -> ("Dynamic Data Type"=w348:dynamicdata)  [unwired: 3 in]
            n156 = Build Cluster Array(w363, w437) -> (→"Parent: R vs Vg : TimeGraph":cluster{dbl, dbl}[])
            n157 = call "Convert to Dynamic Data3"("Array"=w437) -> ("Dynamic Data Type"=w436:dynamicdata)  [unwired: 3 in]
            n158 = Build Cluster Array(w363, w435) -> (→"Parent: Theta vs Vg : TimeGraph":cluster{dbl, "Theta-Value":dbl}[])
            n159 = call "Convert to Dynamic Data4"("Array"=w435) -> ("Dynamic Data Type"=w434:dynamicdata)  [unwired: 3 in]
            n160 = call "R Vs Vg2"("Reset"=FALSE, "Y Input"=w367, "X Input"=w366) -> ("XY Graph"=→"Daughter Resistance vs Vg : XYGraph 2":cluster{"X":dbl[], "Y":dbl[]}[])  [unwired: 7 in, 1 out]
            n161 = Build Cluster Array(w351, w350) -> (→"Temp vs Time: TimeGraph 3":cluster{dbl, "Temperature (K)":dbl}[])
            n162 = Concatenate Strings(w387, w346, w386, w346, w385, w346, w384, w346, w341, w346, "\r\n") -> (w383:string)
            n163 = call "I_leak vs Vg"("Reset"=FALSE, "Y Input"=w438, "X Input"=w366) -> ("XY Graph"=→"I_leak vs Vg : XYGraph":cluster{"X":dbl[], "Y":dbl[]}[])  [unwired: 7 in, 1 out]
            n164 = Format Into String(format string="%.4f", w374) -> (resulting string=w411:string)  [unwired: 2 in, 1 out]
            n165 = Format Into String(format string="%.9f", w406) -> (resulting string=w410:string)  [unwired: 2 in, 1 out]
            n166 = Format Into String(format string="%.12f", w371) -> (resulting string=w409:string)  [unwired: 2 in, 1 out]
            n167 = Format Into String(format string="%.3f", w405) -> (resulting string=w408:string)  [unwired: 2 in, 1 out]
            n168 = call "R Vs Vg"("Reset"=FALSE, "Y Input"=w436, "X Input"=w366) -> ("XY Graph"=→"Parent Resistance vs Vg : XYGraph":cluster{"X":dbl[], "Y":dbl[]}[])  [unwired: 7 in, 1 out]
            n169 = call "Theta Vs Vg"("Reset"=FALSE, "Y Input"=w434, "X Input"=w366) -> ("XY Graph"=→"Parent Theta vs Vg : XYGraph":cluster{"X":dbl[], "Y":dbl[]}[])  [unwired: 7 in, 1 out]
            n170 = Write to Text File(file (use dialog)=w378, text=w383, error in=w376) -> (refnum out=w377:refnum<file>, error out=w375:errorcluster)  [unwired: 1 in, 1 out]
            n171 = Concatenate Strings(w411, w342, w410, w342, w409, w342, w408, w342, w341, w342, "\r\n") -> (w407:string)
            n172 = call "Temp Vs Time"("Reset"=FALSE, "Y Input"=w348, "X Input"=w349) -> ("XY Graph"=→"Temp vs Time : XYGraph 3":cluster{"X":dbl[], "Y":dbl[]}[])  [unwired: 7 in, 1 out]
            n173 = call "Theta Vs Vg2"("Reset"=FALSE, "Y Input"=w365, "X Input"=w366) -> ("XY Graph"=→"Parent Theta vs Vg : XYGraph 2":cluster{"X":dbl[], "Y":dbl[]}[])  [unwired: 7 in, 1 out]
            n174 = Write to Text File(file (use dialog)=w415, text=w407, error in=w414) -> (refnum out=w413:refnum<file>, error out=w412:errorcluster)  [unwired: 1 in, 1 out]
            "Compliance\n Level (A)" <- w395
            "Internal \nMeasurement\nTime" <- w453
          }
        }
        frame True {
          # "Error state for out of bounds"
          n175 = Bundle(cluster=errorcluster {"status"=TRUE, "code"=-1, "source"=""} ("error constant"), "source"="Initial or Final Gate Voltage outside Max/Min bound") -> (w495:errorcluster)  [unwired: 2 in]
          n176 = Select(t=w495, s=w499, f=w498) -> (s? t:f=w494:errorcluster)
        }
      }
    }
  }
  n177 = Close File(refnum=w90, error in=w89) -> (error out=w93:errorcluster)  [unwired: 1 out]
  n178 = call <instrlib>:"Close.vi"("error in (no error)"=w162, "VISA resource name"=w163) -> ("error out"=w161:errorcluster)  [unwired: 9 in]
  n179 = call <instrlib>:"Close.vi"("error in (no error)"=w134, "VISA resource name"=w135) -> ("error out"=w149:errorcluster)  [unwired: 9 in]
  n180 = Close File(refnum=w25, error in=w23) -> (error out=w21:errorcluster)  [unwired: 1 out]
  n181 = call <vilib>:"Simple Error Handler.vi"("error in (no error)"=w161) -> ()  [unwired: 4 in, 5 out]
  n182 = call <vilib>:"Simple Error Handler.vi"("error in (no error)"=w149) -> ()  [unwired: 4 in, 5 out]
  n183 = call <vilib>:"Simple Error Handler.vi"("error in (no error)"=w93) -> ()  [unwired: 4 in, 5 out]
  n184 = call <vilib>:"Simple Error Handler.vi"("error in (no error)"=w21) -> ()  [unwired: 4 in, 5 out]
  "Max/Min(-) \nGate Voltage (V)" <- w105
  "Input Coupling (0: AC)" <- w131
  "External Reference Trigger (0: Sine Zero Crossing)" <- w127
  "Detection Harmonic Number" <- w126
  "Manual Phase (0 Degree)" <- w125
  "Manual Phase (0 Degree) 2" <- w12
  "Detection Harmonic Number 2" <- w10
  "External Reference Trigger (0: Sine Zero Crossing)  2" <- w26
  "Input Coupling (0: AC) 2" <- w11
